vi "COD浓度全局变量.vi"() -> ()   [LabVIEW 2016, in "斯坦道CODMn.lvlib"]
panel:
  in  "基本量程":enum16{"L", "H"}(ring)
  in  "标准液浓度":dbl
  in  "COD浓度（mg/L)":dbl
  # "标准液浓度（mg/L）："
  # "基本量程（20mL可选）："
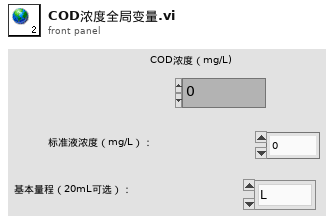
[diagram p1: front panel]
diagram:
